vi "Colour Generater(SubVI).vi"() -> (3 "Colour":enum16{"green", "blue", "red", "yellow"}(ring))   [LabVIEW 2020]
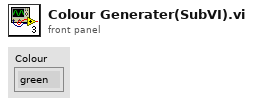
[diagram p1: front panel]
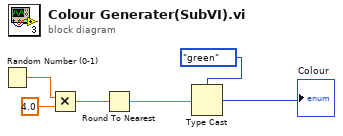
[diagram p0: block diagram]
diagram:
  n1 = Random Number (0-1)() -> (number: 0 to 1=w1:dbl)
  n2 = Multiply(x=w1, y=4.0) -> (x*y=w3:dbl)
  n3 = Round To Nearest(number=w3) -> (nearest integer value=w4:dbl)
  n4 = Type Cast(type=enum16{"green", "blue", "red", "yellow"}."green", x=w4) -> (*(type *) &x=→"Colour":enum16{"green", "blue", "red", "yellow"})
